vi "observacao.vi"() -> ()   [LabVIEW 2012] (continued)
                    n1882 = event-data() -> ()  [unwired: 1 in, 6 out]
                    n1883 = case shown="True" "Go_filtro" {
                      frame False {
                      }
                      frame True {
                        (unwired) "ZERO: Porta serial da CAM1"
                        w2445 = u16 0 items=["ZERO", "AH", "DEC", "TUBO", "CUP"] ("Controlador")
                        n1884 = call "Monta Comando.vi"("Set Point"="Filtro", "Controlador"=w2445) -> ()  [unwired: 5 in, 3 out]
                      }
                    }
                  }
                }
                n1885 = case shown="False" "Velocidade" {
                  tunnel: [TRUE FALSE] -> w2381
                  tunnel: [FALSE TRUE] -> w2380
                  frame False {
                  }
                  frame True {
                  }
                }
                "Rapido" <- w2381
                "Lento" <- w2380
                n1886 = call "Bit Status TUBO.vi"("NomeStatus"=w2395) -> ("StatBit"=w2392:bool)
                n1887 = call "Bit Status TUBO.vi"("NomeStatus"=w2394) -> ("StatBit"=w2391:bool)
                n1888 = call "Bit Status TUBO.vi"("NomeStatus"=w2393) -> ("StatBit"=w2390:bool)
                n1889 = Not(x=w2392) -> (.not. x?=w2401:bool)
                n1890 = And(x=w2392, y=w2391) -> (x .and. y?=w2397:bool)
                "LedRepCam1" <- w2397
                n1891 = Or(x=w2391, y=w2390) -> (x .or. y?=w2402:bool)
                n1892 = And(x=w2392, y=w2390) -> (x .and. y?=w2396:bool)
                "LedCalCam1" <- w2396
                n1893 = property on="SlideCam1" class="Slide (strict)"() -> ("Visible"=w2399:bool)  [unwired: 2 in, 2 out]
                n1894 = Or(x=w2397, y=w2396) -> (x .or. y?=w2400:bool)
                n1895 = And(x=w2401, y=w2402) -> (x .and. y?=w2388:bool)
                n1896 = case shown="True" "Case Constant\n(See Context Help) 10" {
                  frame False {
                  }
                  frame True {
                    w2460 = FALSE
                    w2463 = u16 3 items=["ZERO", "AH", "DEC", "TUBO", "CUP"] ("Controlador")
                    w2461 = u8 0 ("Disabled")
                    n1897 = call "Monta Comando.vi"("Comando"="DESLIGAR", "Dispositivo"="ESP_LAMP", "Controlador"=w2463) -> ()  [unwired: 4 in, 3 out]
                    n1898 = property on="Sent_EspDesvFeixe" class="Bool (strict)"("Disabled"=w2461) -> ()  [unwired: 2 in, 2 out]
                    n1899 = property on="Go_filtro" class="Bool"("Disabled"=w2461) -> ()  [unwired: 2 in, 2 out]
                    n1900 = property on="stopCam1" class="Bool"("Visible"=w2460) -> ()  [unwired: 2 in, 2 out]
                    n1901 = property on="SlideCam1" class="Slide (strict)"("Visible"=w2460) -> ()  [unwired: 2 in, 2 out]
                  }
                }
                n1902 = And(x="Case Constant\n(See Context Help) 10", y=w2388) -> (x .and. y?=w2389:bool)
                n1903 = And(x=w2399, y=w2400) -> (x .and. y?=w2398:bool)
                n1904 = case shown="True" w2389 {
                  frame False {
                  }
                  frame True {
                    w2448 = u8 2 ("Disabled")
                    n1905 = local read "SlideCam1"() -> (w2447:u8)
                    n1906 = Add(x=w2447, y=u8 5) -> (x+y=w2449:u8)
                    n1907 = property on="Sent_EspDesvFeixe" class="Bool (strict)"("Disabled"=w2448) -> ()  [unwired: 2 in, 2 out]
                    n1908 = property on="Go_filtro" class="Bool"("Disabled"=w2448) -> ()  [unwired: 2 in, 2 out]
                    n1909 = Greater Or Equal?(x=w2449, y=u8 100 ("x")) -> (x >= y?=w2451:bool)
                    n1910 = case shown="True" w2451 {
                      selector: w2451 -> [_ w2455]
                      tunnel: w2449 -> [w2453 _]
                      frame False {
                        n1911 = local write "SlideCam1"(w2453) -> ()
                        n1912 = property on="SlideCam1" class="Slide (strict)"("Fill Color"=u32 16750950 ("color(black)")) -> ()  [unwired: 2 in, 2 out]
                      }
                      frame True {
                        n1913 = property on="stopCam1" class="Bool"("Visible"=w2455) -> ()  [unwired: 2 in, 2 out]
                        n1914 = local write "SlideCam1"(u8 90 ("Slide 2")) -> ()
                        n1915 = property on="SlideCam1" class="Slide (strict)"("Fill Color"=u32 16724787 ("color(black)")) -> ()  [unwired: 2 in, 2 out]
                      }
                    }
                  }
                }
                n1916 = case shown="True" w2398 {
                  frame False {
                  }
                  frame True {
                    w2459 = u8 0 ("Disabled")
                    n1917 = property on="Go_filtro" class="Bool"("Disabled"=w2459) -> ()  [unwired: 2 in, 2 out]
                    n1918 = property on="Sent_EspDesvFeixe" class="Bool (strict)"("Disabled"=w2459) -> ()  [unwired: 2 in, 2 out]
                    n1919 = property on="SlideCam1" class="Slide (strict)"("Visible"=FALSE) -> ()  [unwired: 2 in, 2 out]
                  }
                }
              }
              frame "Cam 2" {
                # "Cam 2"
              }
              frame "Cam IV." {
                # "Cam IV"
              }
              frame "Polarim." {
                # "Polarimetro"
              }
              frame "Fotrap" {
                # "Fotrap"
              }
              frame "Coude", Default {
                # "COUDE"
                n1920 = stacked-sequence {
                  frame #0 {
                    w2467 = u16 5 items=["Alarme", "Atencao", "Erro", "Ocupado", "Stop#3", "Cass#3", "MovFoco", "PosSecund", "Mov#2", "Mov#3", "Mov#4", "EspLamp", "HE", "NE", "EspLampRepouso", "EspLampCalibra"] ("NomeStatus")
                    w2466 = u16 7 items=["Alarme", "Atencao", "Erro", "Ocupado", "Stop#3", "Cass#3", "MovFoco", "PosSecund", "Mov#2", "Mov#3", "Mov#4", "EspLamp", "HE", "NE", "EspLampRepouso", "EspLampCalibra"] ("NomeStatus")
                    n1921 = local read "EspAtual"() -> (w2469:string)
                    n1922 = case shown="\"A\"" w2469 {
                      frame "X", Default {
                        w2470 = FALSE
                        n1923 = local write "ledVisivel"(w2470) -> ()
                        n1924 = local write "ledAzul"(w2470) -> ()
                        n1925 = local write "ledVermelho"(w2470) -> ()
                      }
                      frame "M" {
                        w2471 = FALSE
                        n1926 = local write "ledAzul"(w2471) -> ()
                        n1927 = local write "ledVermelho"(w2471) -> ()
                        n1928 = local write "ledVisivel"(w2471) -> ()
                      }
                      frame "A" {
                        # "Espelho A --> Azul\nEspelho B --> Visível\nEspelho C --> Vermelho"
                        n1929 = local write "ledVermelho"(FALSE) -> ()
                        n1930 = local write "ledVisivel"(FALSE) -> ()
                        n1931 = local write "ledAzul"(TRUE) -> ()
                      }
                      frame "B" {
                        # "Espelho A --> Azul\nEspelho B --> Visível\nEspelho C --> Vermelho"
                        n1932 = local write "ledVermelho"(FALSE) -> ()
                        n1933 = local write "ledVisivel"(TRUE) -> ()
                        n1934 = local write "ledAzul"(FALSE) -> ()
                      }
                      frame "C" {
                        # "Espelho A --> Azul\nEspelho B --> Visível\nEspelho C --> Vermelho"
                        n1935 = local write "ledVermelho"(TRUE) -> ()
                        n1936 = local write "ledVisivel"(FALSE) -> ()
                        n1937 = local write "ledAzul"(FALSE) -> ()
                      }
                    }
                    n1938 = call "Bit Status TUBO.vi"("NomeStatus"=w2467) -> ("StatBit"=→"Cjto_3":bool)
                    n1939 = call "Bit Status TUBO.vi"("NomeStatus"=w2466) -> ("StatBit"=→"PosSecundario":bool)
                  }
                  frame #1 {
                    w2491 = u16 5 items=["Alarme", "Atencao", "Erro", "Ocupado", "Stop#3", "Cass#3", "MovFoco", "PosSecund", "Mov#2", "Mov#3", "Mov#4", "EspLamp", "HE", "NE", "EspLampRepouso", "EspLampCalibra"] ("NomeStatus")
                    w2496 = u16 8 items=["Alarme", "Atencao", "Erro", "Ocupado", "Stop#3", "Cass#3", "MovFoco", "PosSecund", "Mov#2", "Mov#3", "Mov#4", "EspLamp", "HE", "NE", "EspLampRepouso", "EspLampCalibra"] ("NomeStatus")
                    w2497 = u16 9 items=["Alarme", "Atencao", "Erro", "Ocupado", "Stop#3", "Cass#3", "MovFoco", "PosSecund", "Mov#2", "Mov#3", "Mov#4", "EspLamp", "HE", "NE", "EspLampRepouso", "EspLampCalibra"] ("NomeStatus")
                    w2498 = u16 10 items=["Alarme", "Atencao", "Erro", "Ocupado", "Stop#3", "Cass#3", "MovFoco", "PosSecund", "Mov#2", "Mov#3", "Mov#4", "EspLamp", "HE", "NE", "EspLampRepouso", "EspLampCalibra"] ("NomeStatus")
                    w2509 = u16 4 items=["Alarme", "Atencao", "Erro", "Ocupado", "Stop#3", "Cass#3", "MovFoco", "PosSecund", "Mov#2", "Mov#3", "Mov#4", "EspLamp", "HE", "NE", "EspLampRepouso", "EspLampCalibra"] ("NomeStatus")
                    w2510 = u16 3 items=["Alarme", "Atencao", "Erro", "Ocupado", "Stop#3", "Cass#3", "MovFoco", "PosSecund", "Mov#2", "Mov#3", "Mov#4", "EspLamp", "HE", "NE", "EspLampRepouso", "EspLampCalibra"] ("NomeStatus")
                    # "CJTO#3 EM \nMOVIMENTO"
                    n1940 = local read "PosSecundario"() -> (w2489:bool)
                    n1941 = call "Bit Status TUBO.vi"("NomeStatus"=w2510) -> ("StatBit"=w2485:bool)
                    n1942 = call "Bit Status TUBO.vi"("NomeStatus"=w2496) -> ("StatBit"=w2502:bool)
                    "#2" <- w2502
                    n1943 = call "Bit Status TUBO.vi"("NomeStatus"=w2497) -> ("StatBit"=w2501:bool)
                    "#3" <- w2501
                    n1944 = call "Bit Status TUBO.vi"("NomeStatus"=w2498) -> ("StatBit"=w2500:bool)
                    "#4" <- w2500
                    n1945 = call "Bit Status TUBO.vi"("NomeStatus"=w2491) -> ("StatBit"=w2488:bool)
                    n1946 = call "Bit Status TUBO.vi"("NomeStatus"=w2509) -> ("StatBit"=w2487:bool)
                    n1947 = Not Equal?(x=w2489, y=w2488) -> (x != y?=w2490:bool)
                    n1948 = Not(x=w2487) -> (.not. x?=w2483:bool)
                    n1949 = And(x=w2490, y=w2487) -> (x .and. y?=w2484:bool)
                    n1950 = Compound Arithmetic op=OR(w2502, w2501, w2500) -> (w2499:bool)
                    n1951 = Compound Arithmetic op=OR(w2484, w2483, w2485) -> (w2486:bool)
                    n1952 = property on="PosSecundario" class="Bool (strict)"("Blinking"=w2484) -> ()  [unwired: 2 in, 2 out]
                    n1953 = property on="Cjto_3" class="Bool (strict)"("Blinking"=w2484) -> ()  [unwired: 2 in, 2 out]
                    n1954 = case shown="True" w2486 {
                      tunnel: [T5."Page Enabled" ("Page Enabled State") T5."Page Disabled" ("Page Enabled State")] -> w2481
                      tunnel: [u8 0 ("Disabled") u8 2 ("Disabled")] -> w2495
                      frame False {
                      }
                      frame True {
                      }
                    }
                    n1955 = property on="MENSAGEM" class="Str"("Visible"=w2483, "Blinking"=w2483) -> ()  [unwired: 2 in, 2 out]
                    n1956 = case shown="True" w2499 {
                      tunnel: w2495 -> [w2514 _]
                      tunnel: [w2514 u8 2 ("Disabled")] -> w2494
                      tunnel: [FALSE TRUE] -> w2493
                      tunnel: [FALSE ("Blinking") TRUE ("Blinking")] -> w2492
                      frame False {
                        n1957 = local write "MENSAGEM 2"("EM MOVIMENTO" ("MENSAGEM 2")) -> ()
                      }
                      frame True {
                        n1958 = local read "EndTime"() -> (w2523:u32)
                        n1959 = Tick Count (ms)() -> (millisecond timer value=w2522:u32)
                        n1960 = Subtract(x=w2523, y=w2522) -> (x-y=w2521:u32)
                        n1961 = Divide(x=w2521, y=u32 1000) -> (x/y=w2518:dbl)
                        n1962 = To Unsigned Long Integer(number=w2518) -> (unsigned 32bit integer=w2519:u32)
                        n1963 = Number To Decimal String(number=w2519) -> (decimal integer string=w2516:string)  [unwired: 1 in]
                        n1964 = Concatenate Strings("EM MOVIMENTO " ("MENSAGEM 2"), w2516) -> (w2517:string)
                        n1965 = local write "MENSAGEM 2"(w2517) -> ()
                      }
                    }
                    n1966 = property on="Setup, Pointing & Guiding" class="TabCtl (strict)"() -> ("Pages"=w2482:refnum<vi>[])  [unwired: 2 in, 2 out]
                    n1967 = Index Array(array=w2482, index=4) -> (element=w2505:refnum<vi>)
                    n1968 = Index Array(array=w2482, index=5) -> (element=w2508:refnum<vi>)
                    n1969 = property class="Page"(reference=w2505, "Page Enabled State"=w2481) -> ()  [unwired: 1 in, 2 out]
                    n1970 = property class="Page"(reference=w2508, "Page Enabled State"=w2481) -> ()  [unwired: 1 in, 2 out]
                    n1971 = case shown="False" w2489 {
                      tunnel: [u8 0 ("Disabled") w2529] -> w2504
                      tunnel: w2494 -> [w2527 _]
                      tunnel: [w2527 w2529] -> w2503
                      frame False {
                        # "COUDE"
                      }
                      frame True {
                        w2529 = u8 2 ("Disabled")
                        # "CASS"
                      }
                    }
                    n1972 = property on="MENSAGEM 2" class="Str"("Visible"=w2493, "Blinking"=w2492) -> ()  [unwired: 2 in, 2 out]
                    n1973 = property on="ledAzul" class="Bool (strict)"("Disabled"=w2504) -> ()  [unwired: 2 in, 2 out]
                    n1974 = property on="ledVisivel" class="Bool (strict)"("Disabled"=w2504) -> ()  [unwired: 2 in, 2 out]
                    n1975 = property on="ledVermelho" class="Bool (strict)"("Disabled"=w2504) -> ()  [unwired: 2 in, 2 out]
                    n1976 = property on="Radio Buttons" class="RadioBtnsControl (strict)"("Disabled"=w2504) -> ()  [unwired: 2 in, 2 out]
                    n1977 = property on="#2" class="Bool (strict)"("Disabled"=w2504) -> ()  [unwired: 2 in, 2 out]
                    n1978 = property on="#3" class="Bool (strict)"("Disabled"=w2504) -> ()  [unwired: 2 in, 2 out]
                    n1979 = property on="#4" class="Bool (strict)"("Disabled"=w2504) -> ()  [unwired: 2 in, 2 out]
                    n1980 = property on="Go_Coudé" class="Bool"("Disabled"=w2503) -> ()  [unwired: 2 in, 2 out]
                  }
                  frame #2 {
                    n1981 = case shown="False" "Go_Coudé" {
                      frame False {
                        w2535 = u16 2 items=["Alarme", "Atencao", "Erro", "Ocupado", "Stop#3", "Cass#3", "MovFoco", "PosSecund", "Mov#2", "Mov#3", "Mov#4", "EspLamp", "HE", "NE", "EspLampRepouso", "EspLampCalibra"] ("NomeStatus")
                        w2536 = u16 3 items=["Alarme", "Atencao", "Erro", "Ocupado", "Stop#3", "Cass#3", "MovFoco", "PosSecund", "Mov#2", "Mov#3", "Mov#4", "EspLamp", "HE", "NE", "EspLampRepouso", "EspLampCalibra"] ("NomeStatus")
                        # "TRATA ERROS DO CONTROLADOR"
                        n1982 = call "Bit Status TUBO.vi"("NomeStatus"=w2535) -> ("StatBit"=w2538:bool)
                        n1983 = call "Bit Status TUBO.vi"("NomeStatus"=w2536) -> ("StatBit"=w2540:bool)
                        n1984 = Not(x=w2540) -> (.not. x?=w2539:bool)
                        n1985 = And(x=w2538, y=w2539) -> (x .and. y?=w2537:bool)
                        n1986 = case shown="True" w2537 {
                          frame False {
                          }
                          frame True {
                            w2543 = u16 3 items=["ZERO", "AH", "DEC", "TUBO", "CUP"] ("Controlador")
                            n1987 = call "Monta Comando.vi"("Comando"="ERROS", "Dispositivo"="PROG" ("Comando"), "Controlador"=w2543) -> ()  [unwired: 4 in, 3 out]
                          }
                        }
                      }
                      frame True {
                        w2544 = u16 3 items=["ZERO", "AH", "DEC", "TUBO", "CUP"] ("Controlador")
                        # "Enviar comando de \nmudar Espelho ABC"
                        n1988 = local read "EspAtual"() -> (w2550:string)
                        n1989 = case shown="\"Visível\"" "Radio Buttons" {
                          tunnel: ["C" ("Comando") "A" ("Comando") "B" ("Comando")] -> w2545
                          tunnel: w2550 -> [w2553 w2559 w2564]
                          tunnel: [w2552 w2558 w2565] -> w2547
                          frame "Vermelho" {
                            n1990 = case shown="\"A\"" w2553 {
                              tunnel: [u32 0 u32 60000 u32 35000] -> w2552
                              frame "C", Default {
                              }
                              frame "B" {
                              }
                              frame "A" {
                              }
                            }
                          }
                          frame "Azul", Default {
                            n1991 = case shown="\"C\"" w2559 {
                              tunnel: [u32 0 u32 35000 u32 60000] -> w2558
                              frame "A", Default {
                              }
                              frame "B" {
                              }
                              frame "C" {
                              }
                            }
                          }
                          frame "Visível" {
                            n1992 = case shown="\"C\"" w2564 {
                              tunnel: [u32 0 u32 60000 u32 35000] -> w2565
                              frame "B", Default {
                              }
                              frame "A" {
                              }
                              frame "C" {
                              }
                            }
                          }
                        }
                        n1993 = Tick Count (ms)() -> (millisecond timer value=w2549:u32)
                        n1994 = Add(x=w2549, y=w2547) -> (x+y=→"EndTime":u32)
                        n1995 = call "Monta Comando.vi"("Comando"=w2545, "Dispositivo"="ESPELHO" ("Comando"), "Controlador"=w2544) -> ()  [unwired: 4 in, 3 out]
                      }
                    }
                  }
                  frame #3 {
                    w2576 = 360.0
                    w2581 = 6.283185307179586
                    n1996 = global read "Global_Telescopio.vi" "guide_ang"() -> (w2591:string)
                    n1997 = global read "Global_Telescopio.vi" "guide_nor"() -> (w2592:string)
                    n1998 = global read "Global_Telescopio.vi" "AH_now"() -> (w2588:dbl)
                    n1999 = global read "Global_Telescopio.vi" "delta_now"() -> (w2589:dbl)
                    n2000 = Add(x=w2588, y=w2589) -> (x+y=w2580:dbl)
                    n2001 = Fract/Exp String To Number(string=w2591) -> (number=w2587:dbl)  [unwired: 3 in, 1 out]
                    n2002 = Fract/Exp String To Number(string=w2592) -> (number=w2590:dbl)  [unwired: 3 in, 1 out]
                    n2003 = Quotient & Remainder(x=w2580, y=w2581) -> (x-y*floor(x/y)=w2583:dbl)  [unwired: 1 out]
                    n2004 = Add(x=w2587, y=w2590) -> (x+y=w2572:dbl)
                    n2005 = Less Than 0?(x=w2583) -> (x < 0?=w2585:bool)
                    n2006 = case shown="True" w2585 {
                      tunnel: w2583 -> [w2593 w2596]
                      tunnel: [w2593 w2594] -> w2582
                      tunnel: w2581 -> [_ w2595]
                      frame False {
                      }
                      frame True {
                        n2007 = Add(x=w2596, y=w2595) -> (x+y=w2594:dbl)
                      }
                    }
                    n2008 = Add(x=124.0, y=w2572) -> (x+y=w2571:dbl)
                    n2009 = Multiply(x=w2582, y=57.29577951 ("x*y")) -> (x*y=w2579:dbl)
                    n2010 = Subtract(x=98.2, y=w2579) -> (x-y=w2578:dbl)
                    n2011 = Add(x=w2571, y=w2578) -> (x+y=w2575:dbl)
                    n2012 = Quotient & Remainder(x=w2575, y=w2576) -> (floor(x/y)=w2577:dbl)  [unwired: 1 out]
                    n2013 = Multiply(x=w2577, y=w2576) -> (x*y=w2574:dbl)
                    n2014 = Subtract(x=w2575, y=w2574) -> (x-y=→"Ang. Fenda":dbl)
                  }
                  frame #4 {
                    # "90"
                    # "270"
                    # "180"
                    # "0"
                    n2015 = event shown="[0] Timeout" {
                      selector: _ -> [_ _ _ _ _ _ _ _ _ _ _]
                      dyn-events: _ -> [_ _ _ _ _ _ _ _ _ _ _]
                      timeout: 10 -> [_ _ _ _ _ _ _ _ _ _ _]
                      event Timeout {
                        n2016 = event-data() -> ()  [unwired: 1 in, 2 out]
                        n2017 = stacked-sequence {
                          frame #0 {
                            n2018 = local read "parou 3"() -> (w2598:bool)
                            n2019 = case shown="True" w2598 {
                              frame False {
                              }
                              frame True {
                                n2020 = call "InstrumentControl.vi"("Input Message"="COUDE REDE POSICAO") -> ("Output Message"=w2601:string)  [unwired: 9 in, 1 out]
                                "Output Message" <- w2601
                                n2021 = Decimal String To Number(string=w2601) -> (number=w2600:i32)  [unwired: 2 in, 1 out]
                                n2022 = while {
                                shift-right: [w2604] -> w2599
                                shift-left: _ -> [w2608]
                                tunnel: w2600 -> [w2604]
                                stop <- TRUE stop-if-true
                                n2023 = Subtract(x=w2608, y=w2604) -> (x-y=w2607:i32)
                                n2024 = Absolute Value(x=w2607) -> (abs(x)=w2606:i32)
                                n2025 = Greater Or Equal?(x=w2606, y=1) -> (x >= y?=→"parou 3":bool)
                                }
                                "Posição Rede" <- w2599
                              }
                            }
                          }
                          frame #1 {
                            n2026 = local read "parou"() -> (w2611:bool)
                            n2027 = local read "parou 2"() -> (w2610:bool)
                            n2028 = case shown="True" w2610 {
                              frame False {
                              }
                              frame True {
                                # "Cada volta -> 10mm\nCada volta -> 4000counts\n1 count = 0,0025mm"
                                n2029 = call "InstrumentControl.vi"("Input Message"="COUDE ESPELHO POSICAO") -> ("Output Message"=w2618:string)  [unwired: 9 in, 1 out]
                                n2030 = Fract/Exp String To Number(string=w2618) -> (number=w2617:dbl)  [unwired: 3 in, 1 out]
                                n2031 = while {
                                shift-right: [w2630] -> w2613
                                shift-left: _ -> [w2631]
                                tunnel: w2617 -> [w2630]
                                tunnel: [w2626] -> w2612
                                stop <- TRUE stop-if-true
                                n2032 = Subtract(x=w2631, y=w2630) -> (x-y=w2629:dbl)
                                n2033 = Absolute Value(x=w2629) -> (abs(x)=w2628:dbl)
                                n2034 = Greater Or Equal?(x=w2628, y=0.02) -> (x >= y?=w2626:bool)
                                "parou 2" <- w2626
                                }
                                "Posição Espelho" <- w2613
                                n2035 = case shown="False" w2612 {
                                frame False {
                                n2036 = call "InstrumentControl.vi"("Input Message"="COUDE SERIAL CHAVEAR OFF") -> ()  [unwired: 9 in, 2 out]
                                }
                                frame True {
                                }
                                }
                                n2037 = Absolute Value(x=w2613) -> (abs(x)=w2614:dbl)
                                n2038 = Less Or Equal?(x=w2614, y=0.5) -> (x <= y?=w2616:bool)
                                n2039 = case shown="False" w2616 {
                                tunnel: w2614 -> [w2623 _]
                                frame False {
                                n2040 = Greater Or Equal?(x=w2623, y=34.5) -> (x >= y?=w2621:bool)
                                n2041 = case shown="True" w2621 {
                                frame False {
                                }
                                frame True {
                                n2042 = local write "Boolean"(TRUE ("Boolean")) -> ()
                                }
                                }
                                }
                                frame True {
                                n2043 = local write "Boolean"(FALSE ("Boolean")) -> ()
                                }
                                }
                              }
                            }
                            n2044 = case shown="True" w2611 {
                              frame False {
                              }
                              frame True {
                                n2045 = call "InstrumentControl.vi"("Input Message"="COUDE FENDA POSICAO") -> ("Output Message"=w2638:string)  [unwired: 9 in, 1 out]
                                n2046 = Fract/Exp String To Number(string=w2638) -> (number=w2637:dbl)  [unwired: 3 in, 1 out]
                                n2047 = Multiply(x=w2637, y=1000.0) -> (x*y=w2635:dbl)
                                n2048 = while {
                                shift-right: [w2645] -> w2634
                                shift-left: _ -> [w2646]
                                tunnel: w2635 -> [w2645]
                                tunnel: [w2641] -> w2633
                                stop <- TRUE stop-if-true
                                n2049 = Subtract(x=w2646, y=w2645) -> (x-y=w2644:dbl)
                                n2050 = Absolute Value(x=w2644) -> (abs(x)=w2643:dbl)
                                n2051 = Greater Or Equal?(x=w2643, y=1.0) -> (x >= y?=w2641:bool)
                                "parou" <- w2641
                                }
                                "Largura da Fenda 2" <- w2634
                                n2052 = case shown="False" w2633 {
                                frame False {
                                n2053 = call "InstrumentControl.vi"("Input Message"="COUDE SERIAL CHAVEAR OFF") -> ()  [unwired: 9 in, 2 out]
                                }
                                frame True {
                                }
                                }
                              }
                            }
                          }
                        }
                      }
                      event "Cathode": Value Change {
                        n2054 = event-data() -> ("NewVal"=w2648:bool)  [unwired: 1 in, 4 out]
                        n2055 = case shown="True" w2648 {
                          frame False {
                          }
                          frame True {
                            n2056 = flat-sequence {
                              frame #0 {
                                w2650 = FALSE ("NeAr")
                                n2057 = local write "Neon"(w2650) -> ()
                                n2058 = local write "Incand"(w2650) -> ()
                                n2059 = local write "Position"("Moving" ("Prisma Position")) -> ()
                                n2060 = call "Comando_Quick_Silver.vi"("COMANDO COMPLETO"="COUDE PRISMA MOVER 0" ("Input Message")) -> ()  [unwired: 2 in, 3 out]
                                n2061 = local write "IronArc"(w2650) -> ()
                              }
                              frame #1 {
                                n2062 = Wait (ms)(milliseconds to wait=u32 50) -> ()  [unwired: 1 out]
                              }
                              frame #2 {
                                n2063 = local write "Position"("Cathode" ("Prisma Position")) -> ()
                              }
                            }
                          }
                        }
                      }
                      event "Neon": Value Change {
                        n2064 = event-data() -> ("NewVal"=w2654:bool)  [unwired: 1 in, 4 out]
                        n2065 = case shown="True" w2654 {
                          frame False {
                          }
                          frame True {
                            n2066 = flat-sequence {
                              frame #0 {
                                w2656 = FALSE ("ThAr")
                                n2067 = local write "Cathode"(w2656) -> ()
                                n2068 = local write "Incand"(w2656) -> ()
                                n2069 = local write "Position"("Moving" ("Prisma Position")) -> ()
                                n2070 = call "Comando_Quick_Silver.vi"("COMANDO COMPLETO"="COUDE PRISMA MOVER 180" ("Input Message")) -> ()  [unwired: 2 in, 3 out]
                                n2071 = local write "IronArc"(w2656) -> ()
                              }
                              frame #1 {
                                n2072 = Wait (ms)(milliseconds to wait=u32 50) -> ()  [unwired: 1 out]
                              }
                              frame #2 {
                                n2073 = local write "Position"("Neon" ("Prisma Position")) -> ()
                              }
                            }
                          }
                        }
                      }
                      event "Incand": Value Change {
                        n2074 = event-data() -> ("NewVal"=w2660:bool)  [unwired: 1 in, 4 out]
                        n2075 = case shown="True" w2660 {
                          frame False {
                          }
                          frame True {
                            n2076 = flat-sequence {
                              frame #0 {
                                w2662 = FALSE ("ThAr")
                                n2077 = local write "Cathode"(w2662) -> ()
                                n2078 = local write "Neon"(w2662) -> ()
                                n2079 = local write "Position"("Moving" ("Prisma Position")) -> ()
                                n2080 = call "Comando_Quick_Silver.vi"("COMANDO COMPLETO"="COUDE PRISMA MOVER 270 " ("Input Message")) -> ()  [unwired: 2 in, 3 out]
                                n2081 = local write "IronArc"(w2662) -> ()
                              }
                              frame #1 {
                                n2082 = Wait (ms)(milliseconds to wait=u32 50) -> ()  [unwired: 1 out]
                              }
                              frame #2 {
                                n2083 = local write "Position"("Incand" ("Prisma Position")) -> ()
                              }
                            }
                          }
                        }
                      }
                      event Value Change {
                        n2084 = event-data() -> ("NewVal"=w2666:T4)  [unwired: 1 in, 4 out]
                        n2085 = case shown="True" w2666 {
                          frame False {
                          }
                          frame True {
                            n2086 = call "InstrumentControl.vi"("Input Message"="COUDE FENDA INICIAR") -> ()  [unwired: 9 in, 2 out]
                          }
                        }
                      }
                      event Value Change {
                        n2087 = event-data() -> ("NewVal"=w2668:T4)  [unwired: 1 in, 4 out]
                        n2088 = case shown="True" w2668 {
                          frame False {
                          }
                          frame True {
                            n2089 = call "Comando_Quick_Silver.vi"("COMANDO COMPLETO"="COUDE ESPELHO INICIAR" ("Input Message")) -> ()  [unwired: 2 in, 3 out]
                          }
                        }
                      }
                      event Value Change {
                        n2090 = event-data() -> ("NewVal"=w2670:T4)  [unwired: 1 in, 4 out]
                        n2091 = case shown="True" w2670 {
                          frame False {
                          }
                          frame True {
                            n2092 = call "InstrumentControl.vi"("Input Message"="COUDE PRISMA INICIAR") -> ()  [unwired: 9 in, 2 out]
                          }
                        }
                      }
                      event "Go Angulo de Difração": Value Change {
                        n2093 = event-data() -> ("NewVal"=w2672:bool)  [unwired: 1 in, 4 out]
                        n2094 = case shown="True" w2672 {
                          frame False {
                          }
                          frame True {
                            # "Envia comando para rede de difração"
                            n2095 = Number To Decimal String(number="Angulo da rede de difração") -> (decimal integer string=w2674:string)  [unwired: 1 in]
                            n2096 = Concatenate Strings("COUDE REDE MOVER ", w2674) -> (w2677:string)
                            n2097 = call "InstrumentControl.vi"("Input Message"=w2677) -> ()  [unwired: 9 in, 2 out]
                            n2098 = local write "parou 3"(TRUE ("parou 3")) -> ()
                          }
                        }
                      }
                      event "Go Largura da Fenda": Value Change {
                        n2099 = event-data() -> ("NewVal"=w2678:bool)  [unwired: 1 in, 4 out]
                        n2100 = case shown="True" w2678 {
                          frame False {
                          }
                          frame True {
                            n2101 = call "InstrumentControl.vi"("Input Message"="COUDE SERIAL CHAVEAR ON") -> ("error out"=w2680:errorcluster)  [unwired: 9 in, 1 out]
                            n2102 = Divide(x="Largura da Fenda", y=1000.0) -> (x/y=w2688:dbl)
                            n2103 = Number To Fractional String(use system decimal point (T)=FALSE, number=w2688, precision (6)=i16 6) -> (F-format string=w2682:string)  [unwired: 1 in]
                            n2104 = Concatenate Strings("COUDE FENDA MOVER ", w2682) -> (w2684:string)
                            n2105 = local write "parou"(TRUE ("parou")) -> ()
                            n2106 = call "InstrumentControl.vi"("error"=w2680, "Input Message"=w2684) -> ()  [unwired: 8 in, 2 out]
                          }
                        }
                      }
                      event "Prisma das Lâmpadas": Value Change {
                        n2107 = event-data() -> ("NewVal"=w2699:bool)  [unwired: 1 in, 4 out]
                        n2108 = case shown="False" w2699 {
                          tunnel: [0.0 ("y") 35.0 ("y")] -> w2697
                          frame False {
                            n2109 = local write "Boolean"(TRUE ("Boolean")) -> ()
                          }
                          frame True {
                            n2110 = local write "Boolean"(FALSE ("Boolean 2")) -> ()
                          }
                        }
                        n2111 = call "InstrumentControl.vi"("Input Message"="COUDE SERIAL CHAVEAR ON") -> ("error out"=w2691:errorcluster)  [unwired: 9 in, 1 out]
                        n2112 = local write "parou 2"(TRUE ("parou 2")) -> ()
                        n2113 = Number To Fractional String(use system decimal point (T)=FALSE, number=w2697, precision (6)=i16 6) -> (F-format string=w2692:string)  [unwired: 1 in]
                        n2114 = Concatenate Strings("COUDE ESPELHO MOVER ", w2692) -> (w2694:string)
                        n2115 = call "InstrumentControl.vi"("error"=w2691, "Input Message"=w2694) -> ()  [unwired: 8 in, 2 out]
                      }
                      event "IronArc": Value Change {
                        n2116 = event-data() -> ("NewVal"=w2704:bool)  [unwired: 1 in, 4 out]
                        n2117 = case shown="True" w2704 {
                          frame False {
                          }
                          frame True {
                            n2118 = flat-sequence {
                              frame #0 {
                                w2706 = FALSE ("ThAr")
                                n2119 = local write "Cathode"(w2706) -> ()
                                n2120 = local write "Neon"(w2706) -> ()
                                n2121 = local write "Position"("Moving" ("Prisma Position")) -> ()
                                n2122 = call "Comando_Quick_Silver.vi"("COMANDO COMPLETO"="COUDE PRISMA MOVER 90 " ("Input Message")) -> ()  [unwired: 2 in, 3 out]
                                n2123 = local write "Incand"(w2706) -> ()
                              }
                              frame #1 {
                                n2124 = Wait (ms)(milliseconds to wait=u32 50) -> ()  [unwired: 1 out]
                              }
                              frame #2 {
                                n2125 = local write "Position"("IronArc" ("Prisma Position")) -> ()
                              }
                            }
                          }
                        }
                      }
                    }
                  }
                }
              }
            }
          }
          frame "FOCUS" {
            # "alterado 23/07/2018"
            # "Modificar e testar TX FOCUS - FOCO\nmudando o VI MONTA CMD FOCO de\ndentro desse VI para o VI MONTA\nCOMMAND utilizado normalmente."
            n2126 = event shown="[2] \"Focus +\": Value Change" {
              selector: _ -> [_ _ _]
              dyn-events: _ -> [_ _ _]
              timeout: 10 -> [_ _ _]
              event Timeout {
                n2127 = event-data() -> ()  [unwired: 1 in, 2 out]
              }
              event "Focus -": Value Change {
                n2128 = event-data() -> ()  [unwired: 1 in, 2 out]
                n2129 = case shown="True" "Focus -" {
                  selector: "Focus -" -> [_ w2764]
                  tunnel: ["stop" ("Comando") "in" ("Comando")] -> w2758
                  tunnel: [u8 0 ("Disabled") u8 2 ("Disabled")] -> w2757
                  frame False {
                  }
                  frame True {
                    n2130 = Not(x=w2764) -> (.not. x?=w2765:bool)
                    n2131 = local write "Focus +"(w2765) -> ()
                  }
                }
                n2132 = property on="GO" class="Bool"("Disabled"=w2757) -> ()  [unwired: 2 in, 2 out]
                n2133 = call "TX focus FOCO.vi"("Comando"=w2758) -> ()  [unwired: 12 in, 3 out]
              }
              event "Focus +": Value Change {
                n2134 = event-data() -> ()  [unwired: 1 in, 3 out]
                n2135 = case shown="True" "Focus +" {
                  selector: "Focus +" -> [_ w2773]
                  tunnel: ["stop" ("Comando") "out" ("Comando")] -> w2767
                  tunnel: [u8 0 ("Disabled") u8 2 ("Disabled")] -> w2766
                  frame False {
                  }
                  frame True {
                    n2136 = Not(x=w2773) -> (.not. x?=w2774:bool)
                    n2137 = local write "Focus -"(w2774) -> ()
                  }
                }
                n2138 = property on="GO" class="Bool"("Disabled"=w2766) -> ()  [unwired: 2 in, 2 out]
                n2139 = call "TX focus FOCO.vi"("Comando"=w2767) -> ()  [unwired: 12 in, 3 out]
              }
            }
            n2140 = case shown="True" "SetDefaultFocus" {
              frame False {
              }
              frame True {
                n2141 = global read "Global_Telescopio.vi" "Foco Instrumento"() -> (w2756:string)
                n2142 = Fract/Exp String To Number(string=w2756) -> (number=w2755:dbl)  [unwired: 3 in, 1 out]
                n2143 = local write "Setpoint"(w2755) -> ()
              }
            }
            n2144 = case shown="True" "GO" {
              tunnel: ["pos" ("Comando") "pos" ("Comando")] -> w2725
              frame False {
              }
              frame True {
                # "inserido para corrigir bug do 10\ndo controlador, 10 --> 9"
                n2145 = control-ref of="GO"() -> (w2788:refnum<vi>)
                n2146 = flat-sequence {
                  tunnel: "Setpoint" -> [w2790]
                  tunnel: [w2795] -> w2782
                  tunnel: w2782 -> [w2800]
                  tunnel: [w2800] -> w2781
                  frame #0 {
                    n2147 = Subtract(x=w2790, y="Phx") -> (x-y=w2794:dbl)
                    n2148 = Less Than 0?(x=w2794) -> (x < 0?=w2792:bool)
                    n2149 = Absolute Value(x=w2794) -> (abs(x)=w2798:dbl)
                    n2150 = Equal?(x=w2798, y=10.0) -> (x = y?=w2796:bool)
                    n2151 = Increment(x=w2790) -> (x+1=w2793:dbl)
                    n2152 = Decrement(x=w2790) -> (x-1=w2791:dbl)
                    n2153 = Select(t=w2793, s=w2792, f=w2791) -> (s? t:f=w2789:dbl)
                    n2154 = Select(t=w2789, s=w2796, f=w2790) -> (s? t:f=w2795:dbl)
                  }
                  frame #1 {
                    n2155 = local write "Phx"(w2800) -> ()
                  }
                }
                n2156 = call "troca nome.vi"("GO"=w2788) -> ("acionou GO"=w2787:bool)
                n2157 = case shown="True" w2787 {
                  tunnel: [u32 6618880 ("real") u32 14453248 ("destino")] -> w2784
                  tunnel: [u8 0 ("Disabled") u8 2 ("Disabled")] -> w2780
                  tunnel: w2788 -> [_ _]
                  tunnel: ["stop" ("Comando") "go" ("Comando")] -> w2786
                  frame False {
                    # "acionou botão STOP"
                  }
                  frame True {
                    # "acionou botão GO"
                    n2158 = call "TX focus FOCO.vi"("Comando"="def", "Setpoint"=20.0) -> ()  [unwired: 11 in, 3 out]
                  }
                }
                n2159 = property on="Foco" class="Slide (strict)"("Fill Color"=w2784) -> ()  [unwired: 2 in, 2 out]
                n2160 = property on="Setpoint" class="DigNum (strict)"("Disabled"=w2780) -> ()  [unwired: 2 in, 2 out]
                n2161 = property on="Focus +" class="Bool (strict)"("Disabled"=w2780) -> ()  [unwired: 2 in, 2 out]
                n2162 = property on="Focus -" class="Bool (strict)"("Disabled"=w2780) -> ()  [unwired: 2 in, 2 out]
                n2163 = call "TX focus FOCO.vi"("Comando"=w2786, "Setpoint"=w2781) -> ()  [unwired: 11 in, 3 out]
                n2164 = property on="minus" class="Bool"("DisabledEnum"=w2780) -> ()  [unwired: 2 in, 2 out]
                n2165 = property on="plus" class="Bool"("DisabledEnum"=w2780) -> ()  [unwired: 2 in, 2 out]
                n2166 = property on="SetDefaultFocus" class="Bool"("DisabledEnum"=w2780) -> ()  [unwired: 2 in, 2 out]
              }
            }
            n2167 = Or(x="minus", y="plus") -> (x .or. y?=w2723:bool)
            n2168 = case shown="True" w2723 {
              tunnel: "minus" -> [_ w2746]
              frame False {
              }
              frame True {
                n2169 = flat-sequence {
                  tunnel: w2746 -> [w2749]
                  frame #0 {
                    n2170 = case shown="False" w2749 {
                      tunnel: ["out" ("Comando") "in" ("Comando")] -> w2748
                      frame False {
                      }
                      frame True {
                      }
                    }
                    n2171 = property on="GO" class="Bool"("Disabled"=u8 2) -> ()  [unwired: 2 in, 2 out]
                    n2172 = call "TX focus FOCO.vi"("Comando"=w2748) -> ()  [unwired: 12 in, 3 out]
                  }
                  frame #1 {
                    n2173 = Wait (ms)(milliseconds to wait=u32 30) -> ()  [unwired: 1 out]
                  }
                  frame #2 {
                    n2174 = property on="GO" class="Bool"("Disabled"=u8 0) -> ()  [unwired: 2 in, 2 out]
                    n2175 = call "TX focus FOCO.vi"("Comando"="stop") -> ()  [unwired: 12 in, 3 out]
                  }
                }
              }
            }
            n2176 = Not(x="GO") -> (.not. x?=w2713:bool)
            n2177 = call "TX focus FOCO.vi"("Comando"=w2725) -> ("pos (deg)"=w2710:dbl, "Parou"=w2711:bool)  [unwired: 12 in, 1 out]
            "On Position" <- w2711
            n2178 = local read "Setpoint"() -> (w2722:dbl)
            n2179 = And(x=w2713, y=w2711) -> (x .and. y?=w2712:bool)
            n2180 = Subtract(x=w2710, y=w2722) -> (x-y=w2721:dbl)
            n2181 = Absolute Value(x=w2721) -> (abs(x)=w2720:dbl)
            n2182 = case shown="True" w2712 {
              tunnel: [w2727 w2738] -> w2715
              tunnel: w2710 -> [w2727 w2729]
              frame False {
                n2183 = Get Date/Time In Seconds() -> (seconds since 1Jan1904=→"x+y":timestamp)
                n2184 = local write "Foco aux"(w2727) -> ()
              }
              frame True {
                w2742 = 8.0 ("y")
                n2185 = Get Date/Time In Seconds() -> (seconds since 1Jan1904=w2731:timestamp)
                n2186 = local read "x+y"() -> (w2734:timestamp)
                n2187 = local read "Foco aux"() -> (w2730:dbl)
                n2188 = Add(x=w2734, y=4.0) -> (x+y=w2732:timestamp)
                n2189 = Less Or Equal?(x=w2731, y=w2732) -> (x <= y?=w2737:bool)
                n2190 = First Call?() -> (First Call?: T/F=w2735:bool)
                n2191 = Or(x=w2737, y=w2735) -> (x .or. y?=w2736:bool)
                n2192 = Add(x=w2730, y=w2742) -> (x+y=w2741:dbl)
                n2193 = Subtract(x=w2730, y=w2742) -> (x-y=w2740:dbl)
                n2194 = case shown="True" w2736 {
                  tunnel: w2729 -> [_ w2743]
                  frame False {
                  }
                  frame True {
                    "Foco aux" <- w2743
                  }
                }
                n2195 = In Range and Coerce(upper limit=w2741, x=w2729, lower limit=w2740) -> (In Range?=w2739:bool)  [unwired: 1 out]
                n2196 = case shown="True" w2739 {
                  tunnel: w2730 -> [_ w2745]
                  tunnel: [w2744 w2745] -> w2738
                  tunnel: w2729 -> [w2744 _]
                  frame False {
                    n2197 = local write "Foco aux"(w2744) -> ()
                  }
                  frame True {
                  }
                }
              }
            }
            n2198 = Less Or Equal?(x=w2720, y=2.0) -> (x <= y?=w2718:bool)
            n2199 = case shown="True" w2718 {
              frame False {
              }
              frame True {
                w2775 = u8 0 ("Disabled")
                # "controlador informa que\nmovimento parou"
                n2200 = control-ref of="GO"() -> (w2776:refnum<vi>)
                n2201 = property on="Setpoint" class="DigNum (strict)"("Disabled"=w2775) -> ()  [unwired: 2 in, 2 out]
                n2202 = property on="Focus +" class="Bool (strict)"("Disabled"=w2775) -> ()  [unwired: 2 in, 2 out]
                n2203 = property on="Focus -" class="Bool (strict)"("Disabled"=w2775) -> ()  [unwired: 2 in, 2 out]
                n2204 = property class="Bool"(reference=w2776, "Boolean Text.Text"="GO") -> ()  [unwired: 1 in, 2 out]
                n2205 = property on="Foco" class="Slide (strict)"("Fill Color"=u32 6618880 ("real")) -> ()  [unwired: 2 in, 2 out]
                n2206 = property on="minus" class="Bool"("DisabledEnum"=w2775) -> ()  [unwired: 2 in, 2 out]
                n2207 = property on="plus" class="Bool"("DisabledEnum"=w2775) -> ()  [unwired: 2 in, 2 out]
                n2208 = property on="SetDefaultFocus" class="Bool"("DisabledEnum"=w2775) -> ()  [unwired: 2 in, 2 out]
              }
            }
            n2209 = local write "Foco"(w2715) -> ()
          }
          frame "ROTATOR" {
            # "MUDANÇA 22/6/11:\nValor default passou a ser carregado no início deste VI."
            n2210 = local read "Default Angle"() -> (w2811:string)
            n2211 = global read "Global_Telescopio.vi" "rotator_def"() -> (w2812:string)
            n2212 = Not Equal?(x=w2812, y=w2811) -> (x != y?=w2810:bool)
            n2213 = case shown="True" "Set Rotator Angle" {
              frame False {
              }
              frame True {
                # "MUDANÇA 22/6/11:\nIncluída a formatação\nda string"
                n2214 = call "Formata_Numeros.vi"("Formato ex-> 7.2"="7.2", "Valor num"="New Angle") -> ("resulting string"=w2818:string)
                "Rotator Angle" <- w2818
                n2215 = global write "Global_Telescopio.vi" "guide_ang"(w2818) -> ()
              }
            }
            n2216 = global write "Global_Telescopio.vi" "Flag-Rotator"(FALSE ("Flag-Rotator")) -> ()
            n2217 = case shown="True" "SetRotatorDefAngle" {
              tunnel: w2811 -> [_ w2816]
              frame False {
              }
              frame True {
                n2218 = local write "Rotator Angle"(w2816) -> ()
                n2219 = global write "Global_Telescopio.vi" "guide_ang"(w2816) -> ()
              }
            }
            n2220 = case shown="True" w2810 {
              tunnel: w2812 -> [_ w2815]
              frame False {
              }
              frame True {
                n2221 = local write "Rotator Angle"(w2815) -> ()
                n2222 = global write "Global_Telescopio.vi" "guide_ang"(w2815) -> ()
                "Default Angle" <- w2815
              }
            }
          }
          frame "DOME" {
            w2833 = u16 6 items=["Alarme", "Atencao", "Erro", "Ocupado", "TBD", "LCB", "Trapeira", "Paravento", "DomoRap", "DomoCW", "DomoCCW", "TBD", "Em movimento", "TBD"] ("NomeStatus")
            w2837 = u16 3 items=["Alarme", "Atencao", "Erro", "Ocupado", "TBD", "LCB", "Trapeira", "Paravento", "DomoRap", "DomoCW", "DomoCCW", "TBD", "Em movimento", "TBD"] ("NomeStatus")
            # "MUDANÇA:\nO CW CCW comandos enviados ao controlador\nde girar e parar, estão escondidos. 26-01-2022"
            # "MUDANÇA:\nO RESET do uC CUP apaga o estado da trapeira (e paravento) o que compromote seu controle.\nNecessário implantar sensor de estado da trapeira."
            n2223 = global read "Global_Telescopio.vi" "Telescopio"() -> (w2828:bool)
            n2224 = local read "StatShutter"() -> (w2836:string)
            n2225 = local read "StatDome"() -> (w2838:string)
            n2226 = call "Bit Status CUP.vi"("NomeStatus"=w2837) -> ("StatBit"=w2834:bool)
            n2227 = Select(t=1, s=w2828, f=2) -> (s? t:f=w2826:i32)
            n2228 = event shown="[4] \"BtShutClose\": Value Change" {
              selector: _ -> [_ _ _ _ _ _ _ _]
              dyn-events: _ -> [_ _ _ _ _ _ _ _]
              timeout: 10 -> [_ _ _ _ _ _ _ _]
              tunnel: [FALSE ("NewVal") w2923 w2940 FALSE ("NewVal") FALSE ("NewVal") _ _ _] -> w2835
              tunnel: w2826 -> [_ w2922 _ _ _ _ _ _]
              event Timeout {
                n2229 = event-data() -> ()  [unwired: 1 in, 2 out]
              }
              event "BtDomeGO": Value Change {
                n2230 = event-data() -> ("NewVal"=w2924:bool)  [unwired: 1 in, 5 out]
                n2231 = local read "StatDome"() -> (w2927:string)
                n2232 = Equal?(x=w2927, y="Stopped" ("Status")) -> (x = y?=w2925:bool)
                n2233 = And(x=w2924, y=w2925) -> (x .and. y?=w2923:bool)
                n2234 = case shown="True" w2923 {
                  tunnel: w2922 -> [_ w2928]
                  frame False {
                  }
                  frame True {
                    n2235 = local read "DomeNewPos"() -> (w2935:i32)
                    n2236 = global read "Global_Telescopio.vi" "ErroMaxCup"() -> (w2932:i16)
                    n2237 = global read "Global_Telescopio.vi" "PosCUP"() -> (w2934:i16)
                    n2238 = Multiply(x=w2935, y=w2928) -> (x*y=w2929:i32)
                    n2239 = Subtract(x=w2929, y=w2934) -> (x-y=w2933:i32)
                    n2240 = Absolute Value(x=w2933) -> (abs(x)=w2931:i32)
                    n2241 = Greater?(x=w2931, y=w2932) -> (0:w2930:bool)
                    n2242 = case shown="True" w2930 {
                      tunnel: w2929 -> [_ w2938]
                      frame False {
                      }
                      frame True {
                        # "Desabilita todas Abas"
                        n2243 = local write "DOME"(FALSE) -> ()
                        n2244 = local write "DestCUP"(w2938) -> ()
                        n2245 = property on="Setup, Pointing & Guiding" class="TabCtl (strict)"("Page Selector Visible"=FALSE) -> ()  [unwired: 2 in, 2 out]
                        n2246 = local write "StatDome"("Not Ready" ("Status")) -> ()
                      }
                    }
                  }
                }
              }
              event "BtDomeSTOP": Value Change {
                n2247 = event-data() -> ("NewVal"=w2940:bool)  [unwired: 1 in, 5 out]
                n2248 = case shown="True" w2940 {
                  frame False {
                  }
                  frame True {
                    n2249 = local read "StatDome"() -> (w2941:string)
                    n2250 = case shown="\"Stopped\", Default" w2941 {
                      frame "Stopped", Default {
                      }
                      frame "Moving" {
                        w2942 = u16 4 items=["ZERO", "AH", "DEC", "TUBO", "CUP"] ("Controlador")
                        n2251 = local write "StatDome"("Stopping" ("Status")) -> ()
                        n2252 = call "Monta Comando.vi"("Comando"="PARAR", "Dispositivo"="PROG", "Controlador"=w2942) -> ()  [unwired: 4 in, 3 out]
                      }
                      frame "Not Ready" {
                        n2253 = local write "StatDome"("Stopped" ("Status")) -> ()
                      }
                    }
                  }
                }
              }
              event "BtShutOpen": Value Change {
                n2254 = event-data() -> ("NewVal"=w2948:bool)  [unwired: 1 in, 5 out]
                n2255 = case shown="True" w2948 {
                  frame False {
                  }
                  frame True {
                    n2256 = local read "StatShutter"() -> (w2949:string)
                    n2257 = case shown="\"Closed\"" w2949 {
                      frame "Opened", Default {
                      }
                      frame "Closed" {
                        w2950 = FALSE ("WeakSel")
                        w2951 = FALSE ("Coude")
                        w2952 = T10."Enabled" ("Disabled")
                        n2258 = property on="Coude" class="Bool (strict)"("DisabledEnum"=w2952) -> ()  [unwired: 2 in, 2 out]
                        n2259 = property on="Weak" class="Bool (strict)"("Disabled"=w2952) -> ()  [unwired: 2 in, 2 out]
                        n2260 = local write "StatShutter"("Busy to Open" ("Status")) -> ()
                        n2261 = property on="Medium" class="Bool (strict)"("Disabled"=w2952) -> ()  [unwired: 2 in, 2 out]
                        n2262 = property on="Strong" class="Bool (strict)"("Disabled"=w2952) -> ()  [unwired: 2 in, 2 out]
                        n2263 = local write "WeakSel"(w2950) -> ()
                        n2264 = local write "MediumSel"(w2950) -> ()
                        n2265 = local write "Coude"(w2951) -> ()
                        n2266 = local write "Weak"(w2951) -> ()
                        n2267 = local write "Medium"(w2951) -> ()
                        n2268 = local write "Strong"(w2951) -> ()
                        n2269 = stacked-sequence {
                          frame #0 {
                            w2955 = u16 4 items=["ZERO", "AH", "DEC", "TUBO", "CUP"] ("Controlador")
                            n2270 = call "Monta Comando.vi"("Comando"="DESLIGAR", "Dispositivo"="FLAT_WEAK", "Controlador"=w2955) -> ()  [unwired: 4 in, 3 out]
                          }
                          frame #1 {
                            w2958 = u16 4 items=["ZERO", "AH", "DEC", "TUBO", "CUP"] ("Controlador")
                            n2271 = call "Monta Comando.vi"("Comando"="DESLIGAR", "Dispositivo"="FLAT_LO", "Controlador"=w2958) -> ()  [unwired: 4 in, 3 out]
                          }
                          frame #2 {
                            w2961 = u16 4 items=["ZERO", "AH", "DEC", "TUBO", "CUP"] ("Controlador")
                            n2272 = call "Monta Comando.vi"("Comando"="DESLIGAR", "Dispositivo"="FLAT_HI", "Controlador"=w2961) -> ()  [unwired: 4 in, 3 out]
                          }
                          frame #3 {
                            w2963 = u16 4 items=["ZERO", "AH", "DEC", "TUBO", "CUP"] ("Controlador")
                            n2273 = call "Monta Comando.vi"("Comando"="DESLIGAR", "Dispositivo"="FLAT_COUDE", "Controlador"=w2963) -> ()  [unwired: 4 in, 3 out]
                          }
                        }
                        n2274 = local write "StrongSel"(w2950) -> ()
                        n2275 = local write "CoudeSel"(w2950) -> ()
                      }
                    }
                  }
                }
              }
              event "BtShutClose": Value Change {
                n2276 = event-data() -> ("NewVal"=w2967:bool)  [unwired: 1 in, 5 out]
                n2277 = case shown="True" w2967 {
                  frame False {
                  }
                  frame True {
                    n2278 = stacked-sequence {
                      frame #0 {
                        # "MUDANÇA:\nRemovido CASE que não setava essas\nvariáveis se StatShutter = Closed para\ngarantir fechamento da Trapeira."
                        n2279 = local write "DOME"(FALSE) -> ()
                        n2280 = local write "StatShutter"("Busy to Close" ("Status")) -> ()
                      }
                      frame #1 {
                        # "Escreve no LOG o estado do shutter"
                        # "Timer para escrever no log\ne enviar comando:\nCUP TRAPEIRA PARAR"
                        n2281 = Tick Count (ms)() -> (millisecond timer value=w2970:u32)
                        n2282 = local write "sendCommandShutter"(TRUE ("writeShutterLog")) -> ()
                        n2283 = local write "shutterTimeOld"(w2970) -> ()
                        n2284 = local write "timeStatShutterAlert"(w2970) -> ()
                        n2285 = call "Log_Shutter.vi"("command"=" ", "domeState"="CLOSED " ("command"), "pathLogDomeFile"="C:\\TCS\\LOG\\SHUTTER\\SHUTTER.TXT" ("pathLogFocoString")) -> ()  [unwired: 6 in]
                      }
                    }
                  }
                }
              }
              event "BtParavUp": Value Change {
                n2286 = event-data() -> ("NewVal"=w2975:bool)  [unwired: 1 in, 5 out]
                n2287 = case shown="True" w2975 {
                  frame False {
                  }
